vi "UpdateGUIFromSeq.vi"(0 "TestSeqClass in":refnum<class "TestSeqClass.lvclass">, 11 "error in (no error)":errorcluster) -> (4 "TestSeqClass out":refnum<class "TestSeqClass.lvclass">, 15 "error out":errorcluster)   [LabVIEW 2017]
uses:
  TestSeqClass.lvclass
  Typedef/TestStatus.ctl
  TestSeqClass.lvclass/TestSeqClass.ctl
  Read CurrentTestPointer.vi
  TestMeasureStep/TestMeasureStep.lvclass
  GUIHandler_Main/GUI_Handler_Main.lvclass
  GUIHandler/GUI_Handler_Seq.lvclass
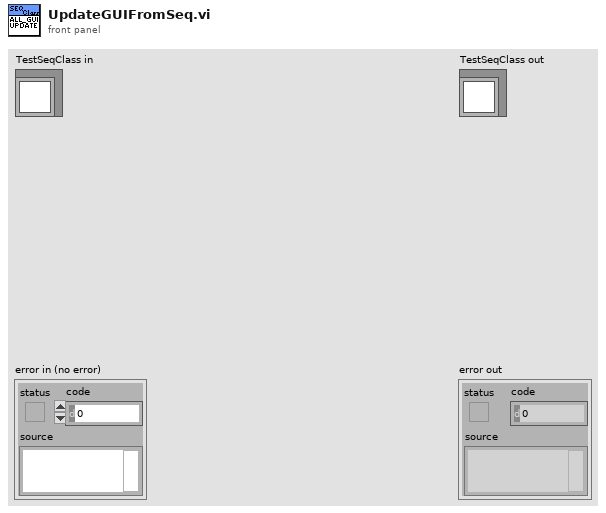
[diagram p1: front panel]
types:
  T1 = typedef "TestStatus.ctl" = enum16{"Not Executed", "Passed", "Failed", "Inconclusive", "Processing"}
  T2 = typedef "TestTypeSelect.ctl" = enum16{"Calibration", "Testing"}
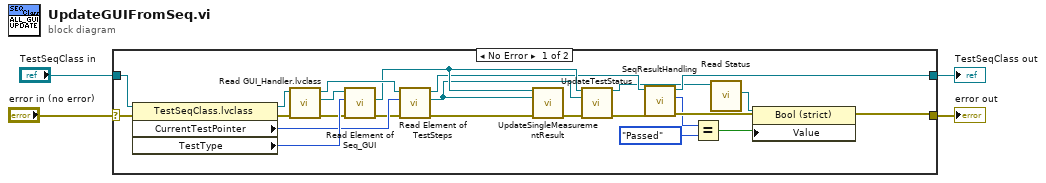
[diagram p0: block diagram]
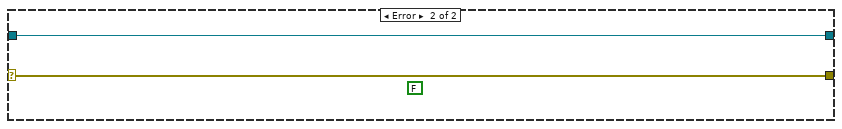
[diagram p2: hidden frame]
diagram:
  n1 = case shown="No Error" "error in (no error)" {
    selector: "error in (no error)" -> [w26 w29]
    tunnel: [w12 w29] -> w3
    tunnel: [w10 w28] -> w1
    tunnel: "TestSeqClass in" -> [w27 w28]
    frame No Error {
      n2 = property class="TestSeqClass.lvclass"(reference=w27, error in=w26) -> (reference out=w25:refnum<class "TestSeqClass.lvclass">, error out=w24:errorcluster, "CurrentTestPointer"=w20:u32, "TestType"=w22:T2)
      n3 = call-dynamic "Read GUI_Handler.lvclass.vi"("error in (no error)"=w24, "TestSeqClass in"=w25) -> ("error out"=w15:errorcluster, "GUI_Handler.lvclass"=w23:refnum<class "GUI_Handler_Main.lvclass">, "TestSeqClass out"=w21:refnum<class "TestSeqClass.lvclass">)  [unwired: 7 in]
      n4 = call-dynamic "Read Element of Seq_GUI.vi"("error in (no error)"=w15, "Variant"=w22, "GUI_Handler_Main in"=w23) -> ("error out"=w14:errorcluster, "GUI_Handler_Seq.lvclass"=w18:refnum<class "GUI_Handler_Seq.lvclass">)  [unwired: 6 in, 1 out]
      n5 = call "Read Element of TestSteps.vi"("error in (no error)"=w14, "index"=w20, "TestSeqClass in"=w21) -> ("error out"=w16:errorcluster, "TestMeasureStep.lvclass"=w17:refnum<class "TestMeasureStep.lvclass">, "TestSeqClass out"=w11:refnum<class "TestSeqClass.lvclass">)  [unwired: 6 in]
      n6 = call "UpdateSingleMeasurementResult.vi"("GUI_Handler_Seq in"=w18, "TestMeasureStep in"=w17, "error in (no error)"=w16) -> ("error out"=w19:errorcluster)  [unwired: 11 in, 1 out]
      n7 = call "UpdateTestStatus.vi"("GUI_Handler_Seq in"=w18, "TestMeasureStep in"=w17, "error in (no error)"=w19) -> ("GUI_Handler_Seq out"=w9:refnum<class "GUI_Handler_Seq.lvclass">, "error out"=w13:errorcluster)  [unwired: 11 in]
      n8 = call "SeqResultHandling.vi"("error in (no error)"=w13, "TestSeqClass in"=w11) -> ("error out"=w12:errorcluster, "OverallTestStatus"=w7:T1, "TestSeqClass out"=w10:refnum<class "TestSeqClass.lvclass">)  [unwired: 7 in]
      n9 = Equal?(x=w7, y=TestStatus."Passed") -> (x = y?=w5:bool)
      n10 = call-dynamic "Read Status.vi"("GUI_Handler_Seq in"=w9) -> ("Status"=w8:refnum<vi>)  [unwired: 8 in, 2 out]
      n11 = property class="Bool (strict)"(reference=w8, "Value"=w5) -> ()  [unwired: 1 in, 2 out]
    }
    frame Error {
      (unwired) FALSE
    }
  }
  "error out" <- w3
  "TestSeqClass out" <- w1
